vi "init.vi"(8 "error in (no error)":errorcluster, 11 "CompactDAQ in":refnum<class "CompactDAQ.lvclass">) -> (0 "error out":errorcluster, 3 "CompactDAQ out":refnum<class "CompactDAQ.lvclass">)   [LabVIEW 2017, in "CompactDAQ.lvclass"]
uses:
  CompactDAQ.lvclass
  <userlib>/Common Components/Hardware/DAQ/DAQ .lvclass
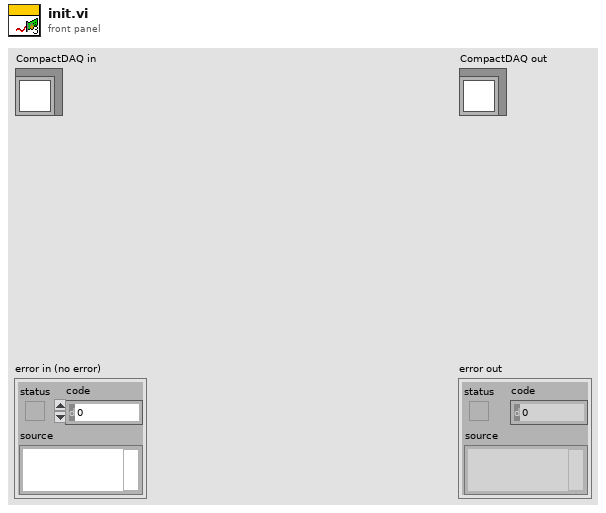
[diagram p1: front panel]
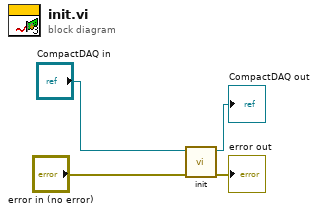
[diagram p0: block diagram]
diagram:
  n1 = call-parent "init.vi"("error in (no error)"="error in (no error)", "DAQ  in"="CompactDAQ in") -> ("error out"=→"error out":errorcluster, "DAQ  out"=→"CompactDAQ out":refnum<class "CompactDAQ.lvclass">)  [unwired: 8 in]
